vi "FTW-File-CompareFilepaths.vi"(0 "Base Path":path, 5 "Path to Compare":path) -> (4 "Relative Path from Base":path, 6 "Common Path":path, 8 "Path relative to Base?":bool)   [LabVIEW 2015]
panel:
  # "Inputs"
  # "Outputs"
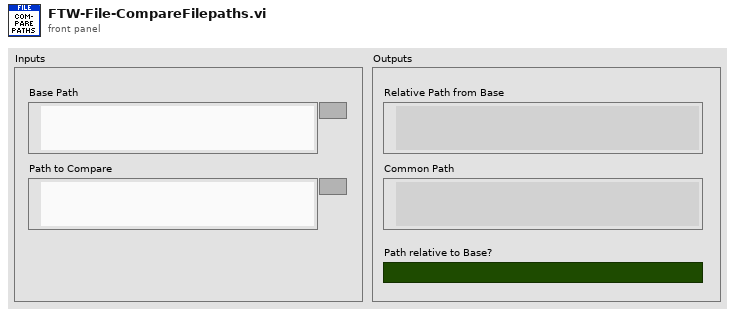
[diagram p1: front panel]
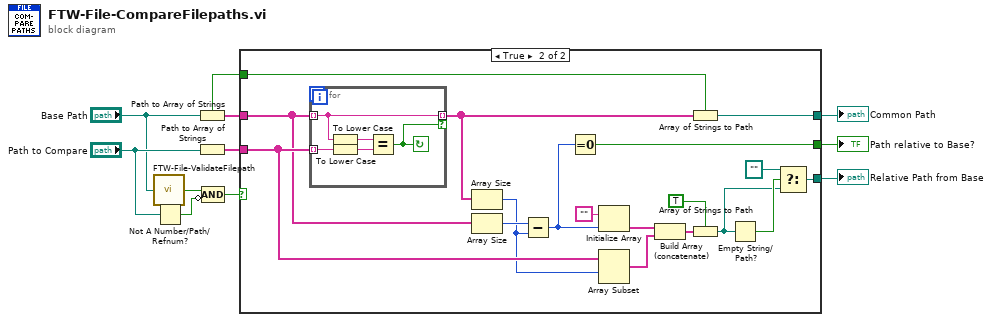
[diagram p0: block diagram]
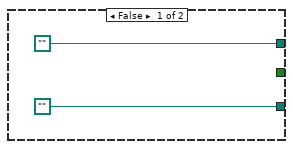
[diagram p2: hidden frame]
diagram:
  n1 = call "FTW-File-ValidateFilepath.vi"("Filepath"="Base Path") -> ("Valid?"=w3:bool)
  n2 = Not A Number/Path/Refnum?(number/path/refnum="Path to Compare") -> (NaN/Path/Refnum?=w6:bool)
  n3 = Path to Array of Strings(0:"Base Path") -> (1:w7:bool, 2:w9:string[])
  n4 = Path to Array of Strings(0:"Path to Compare") -> (2:w8:string[])  [unwired: 1 out]
  n5 = Compound Arithmetic op=AND(w3, invert w6) -> (w5:bool)
  n6 = case shown="True" w5 {
    tunnel: w9 -> [_ w19]
    tunnel: w8 -> [_ w29]
    tunnel: [path "" w31] -> w2
    tunnel: [path "" w22] -> w1
    tunnel: [_ w14] -> w10
    tunnel: w7 -> [_ w20]
    frame False {
    }
    frame True {
      n7 = for {
        tunnel: w19 -> [w33] mode=indexing
        tunnel: w29 -> [w36] mode=indexing
        tunnel: [w33] -> w18 mode=indexing if=w32
        stop <- w32 continue-if-true
        n8 = To Lower Case(string=w33) -> (all lower case string=w35:string)
        n9 = To Lower Case(string=w36) -> (all lower case string=w34:string)
        n10 = Equal?(x=w35, y=w34) -> (x = y?=w32:bool)
      }
      n11 = Array Size(array=w18) -> (size(s)=w17:i32)
      n12 = Array Size(array=w19) -> (size(s)=w26:i32)
      n13 = Subtract(x=w26, y=w17) -> (x-y=w15:i32)
      n14 = Equal To 0?(x=w15) -> (x = 0?=w14:bool)
      n15 = Initialize Array("", w15) -> (w30:string[])
      n16 = Array Subset(array=w29, index=w17) -> (w28:string[])  [unwired: 1 in]
      n17 = Build Array (concatenate)(w30, w28) -> (w27:string[])
      n18 = Array of Strings to Path(0:w18, 1:w20) -> (2:w31:path)
      n19 = Array of Strings to Path(0:w27, 1:TRUE ("relative")) -> (2:w23:path)
      n20 = Empty String/Path?(string/path=w23) -> (empty?=w24:bool)
      n21 = Select(t=path "", s=w24, f=w23) -> (s? t:f=w22:path)
    }
  }
  "Relative Path from Base" <- w1
  "Path relative to Base?" <- w10
  "Common Path" <- w2
